vi "9-1 파일경로.vi"() -> ()   [LabVIEW 2014]
uses:
  <vilib>/Utility/sysdir.llb/System Directory Type.ctl
panel:
  out "에러 출력":errorcluster
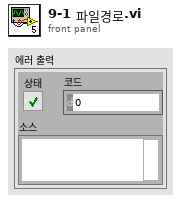
[diagram p1: front panel]
types:
  T1 = enum16{"open", "replace", "create", "open or create", "replace or create", "replace or create with confirmation"}
  T2 = typedef "System Directory Type.ctl" = i32
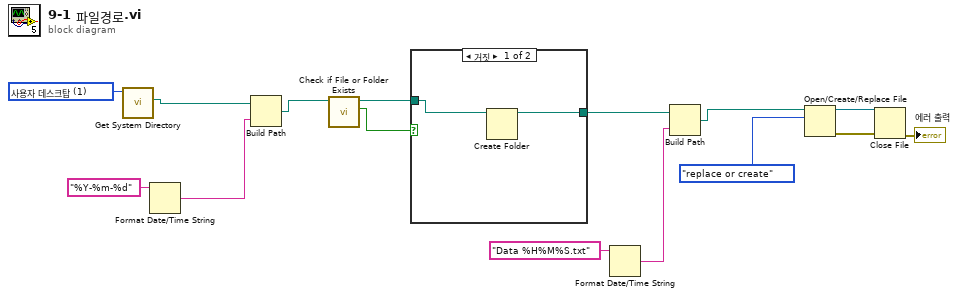
[diagram p0: block diagram]
diagram:
  w15 = T2 1 items=["사용자 홈"=0, "사용자 데스크탑"=1, "사용자 문서"=2, "사용자 어플리케이션 데이터"=3, "사용자 환경"=4, "사용자 임시"=5, "퍼블릭 문서"=6, "퍼블릭 어플리케이션 데이터"=7, "퍼블릭 환경"=8, "퍼블릭 캐시"=13, "시스템 코어 라이브러리"=9, "시스템 설치된 라이브러리"=10, "어플리케이션 파일"=11, "부팅 볼륨 루트"=12] ("system directory type")
  n1 = call <vilib>:"Get System Directory.vi"("system directory type"=w15) -> ("system directory"=w13:path)  [unwired: 10 in]
  n2 = Format Date/Time String(time format string (%c)="%Y-%m-%d" ("시간 포맷 문자열 (%c)")) -> (date/time string=w12:string)  [unwired: 2 in]
  n3 = Build Path(base path=w13, name or relative path=w12) -> (appended path=w11:path)
  n4 = call <vilib>:"Check if File or Folder Exists.vi"("path"=w11) -> ("file or folder exists?"=w9:bool, "dup path"=w10:path)  [unwired: 8 in, 1 out]
  n5 = case shown="거짓" w9 {
    tunnel: w10 -> [w17 w18]
    tunnel: [w16 w18] -> w7
    frame False {
      n6 = Create Folder(path (use dialog)=w17) -> (created path=w16:path)  [unwired: 2 in, 2 out]
    }
    frame True {
    }
  }
  n7 = Format Date/Time String(time format string (%c)="Data %H%M%S.txt" ("시간 포맷 문자열 (%c)")) -> (date/time string=w6:string)  [unwired: 2 in]
  n8 = Build Path(base path=w7, name or relative path=w6) -> (appended path=w5:path)
  n9 = Open/Create/Replace File(file path (use dialog)=w5, operation (0:open)=T1."replace or create" ("동작(0:open)")) -> (refnum out=w3:refnum<file>, error out=w2:errorcluster)  [unwired: 4 in, 1 out]
  n10 = Close File(refnum=w3, error in=w2) -> (error out=→"에러 출력":errorcluster)  [unwired: 1 out]
